vi "Read Observer Array.vi"(8 "error in (no error)":errorcluster, 11 "Subject in":refnum<class "Subject.lvclass">) -> (0 "error out":errorcluster, 2 "Observer Array":refnum<class "Message Enqueuer.lvclass">[](array[class]), 3 "Subject out":refnum<class "Subject.lvclass">)   [LabVIEW 2013, in "Observer Pattern Actor Interface.lvlib" / "Subject.lvclass"]
uses:
  Subject.lvclass
  <vilib>/ActorFramework/Message Enqueuer/Message Enqueuer.lvclass
  Subject.lvclass/Subject.ctl
  Global 2.vi
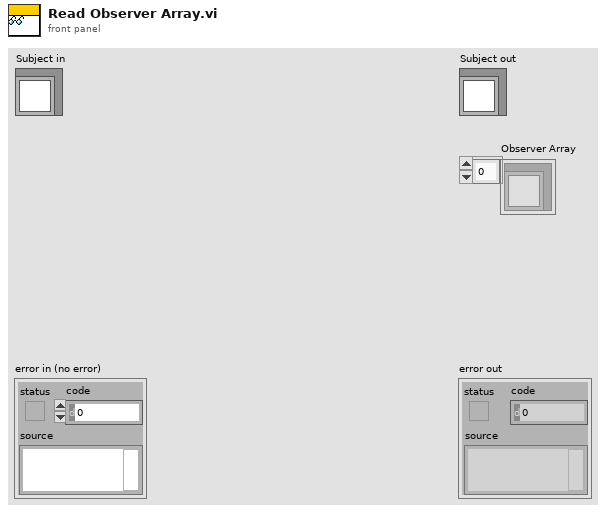
[diagram p1: front panel]
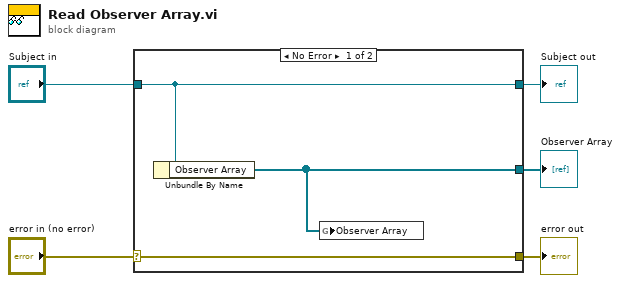
[diagram p0: block diagram]
diagram:
  n1 = case shown="No Error" "error in (no error)" {
    selector: "error in (no error)" -> [w8 w9]
    tunnel: [w8 w9] -> w4
    tunnel: [w7 w10] -> w2
    tunnel: "Subject in" -> [w7 w10]
    tunnel: [w6 _] -> w1
    frame No Error {
      n2 = Unbundle By Name(w7) -> ("Observer Array"=w6:refnum<class "Message Enqueuer.lvclass">[])
      n3 = global write "Global 2.vi" "Observer Array"(w6) -> ()
    }
    frame Error {
    }
  }
  "error out" <- w4
  "Subject out" <- w2
  "Observer Array" <- w1
